vi "TRNPRPdll.vi"(8 "error in (no error)":errorcluster, 11 "Inputs":cluster{"t":dbl, "D":dbl, "z":dbl[]}) -> (0 "error out":errorcluster, 3 "Outputs":T1)   [LabVIEW 2015]
doc: "subroutine TRNPRPdll(t, D, z, eta, tcx, ierr, herr, herr_length)\n\nCompute the transport properties thermal conductivity and viscosity as functions of temperature, density, and\ncomposition.\n\n*** Warning *** Do NOT call this routine for two-phase states, otherwise it will return a metastable state if\nnear the phase boundary or complete nonsense at other conditions. The value of q that is returned from the flash\nroutines will indicate a two phase state by returning a value between 0 and 1. In such a situation, the transport\nproperties can only be calculated for the saturated liquid and vapor states. For example, when calling PHFLSH:\ncall subroutine PHFLSH (P,h,z,T,D,Dl,Dv,x,y,q,e,s,Cv,Cp,w,ierr,herr) If q>0 and q<1, then values of the liquid\ncompositions will be returned in the x and y arrays, and the transport properties of the liquid and vapor states can\nbe calculated as such: call TRNPRP (T,Dl,x,etaliq,tcxliq,ierr,herr) call TRNPRP (T,Dv,y,etavap,tcxvap,ierr,herr)\n\nINPUTS:\nt -- Temperature [K]\nD -- Molar density [mol/L]\nz -- Composition array (array of mole fractions)\n\nOUTPUTS:\neta -- Viscosity [uPa-s]\ntcx -- Thermal conductivity [W/m-K]\nierr -- Error flag: 0 - Successful \n 502 - Unknown viscosity or thermal conductivity model specified \n 503 - One or more inputs are out of bounds for the ECS model \n 504 - Inputs to the vis. and th. cond. correlations are out 2of range \n 540 - Transport equations are not available for one or more of the fluids \n 541 - Transport equations are not available for mixtures with water at molar concentrations greater than 5% \n 542 - Transport equations are not available for mixtures with alcohols \n 543 - Transport equations are not available for the ammonia/water mixture \n -508 - Invalid region for viscosity of reference fluid 1 \n -558 - 2-D Newton-Raphson method for conformal temperature and density did not converge \n -560 - Pure fluid is exactly at the critical point; thermal conductivity is infinite \n 561 - Pure fluid correlation produced an erroneous value for either viscosity or thermal conductivity \n 5## - One or more inputs to the thermal conductivity correlation are out of range; results may be in error \n 5## - One or more inputs to the viscosity correlation are out of range; results may be in error \n 5## - Pure fluid correlation out of range; attempted to use ECS method\nherr -- Error string (character*255)\nherr_length -- length of variable herr (default: 255)"
uses:
  REFPROP.dll
panel:
  # "REFPROP-TRNPRPdll.vi"
  # "void  TRNPRPdll(double *t, double *D, double *z, double *eta, double *tcx, int32_t *ierr, CStr herr, int32_t herr_length)"
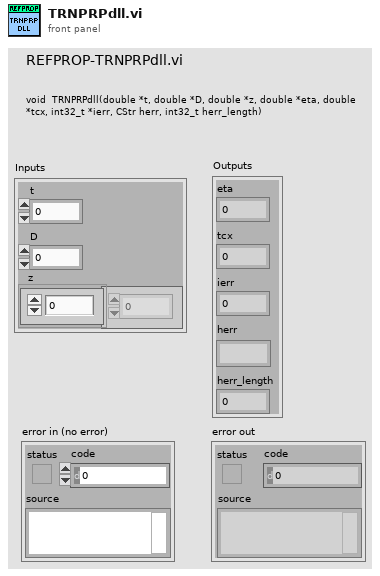
[diagram p1: front panel]
types:
  T1 = cluster{"eta":dbl, "tcx":dbl, "ierr":i32, "herr":string, "herr_length":i32}
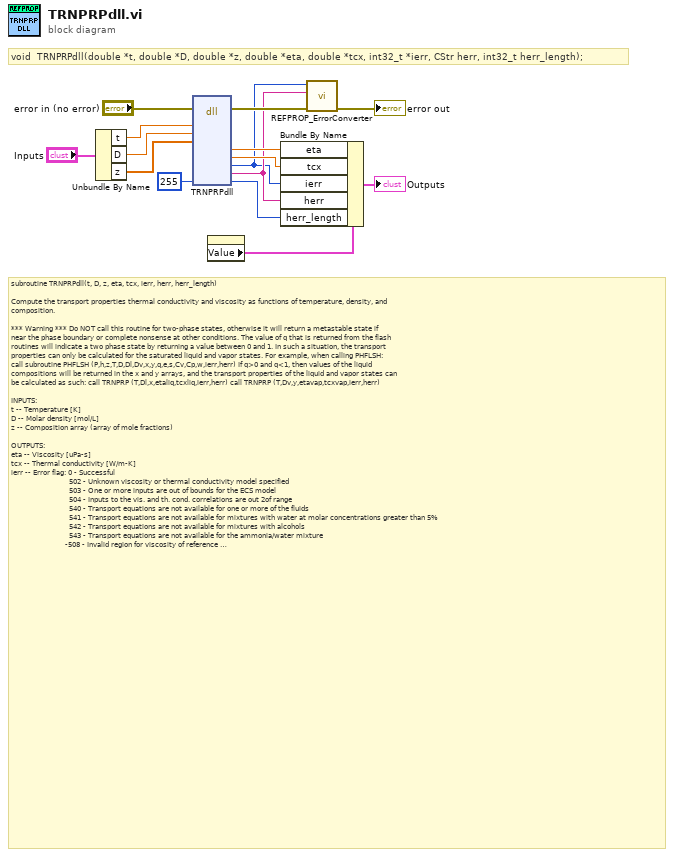
[diagram p0: block diagram]
diagram:
  # "void  TRNPRPdll(double *t, double *D, double *z, double *eta, double *tcx, int32_t *ierr, CStr herr, int32_t herr_length);"
  # "subroutine TRNPRPdll(t, D, z, eta, tcx, ierr, herr, herr_length)\n\nCompute the transport properties thermal conductivity and viscosity as functions of temperature, density, and\ncomposition.\n\n*** Warning *** Do NOT call this routine for two-phase states, otherwise it will return a metastable state if\nnear the phase boundary or complete nonsense at other conditions. The value of q that is returned from the flash\nroutines will indicate a two phase state by returning a value between 0 and 1. In such a situation, the transport\nproperties can only be calculated for the saturated liquid and vapor states. For example, when calling PHFLSH:\ncall subroutine PHFLSH (P,h,z,T,D,Dl,Dv,x,y,q,e,s,Cv,Cp,w,ierr,herr) If q>0 and q<1, then values of the liquid\ncompositions will be returned in the x and y arrays, and the transport properties of the liquid and vapor states can\nbe calculated as such: call TRNPRP (T,Dl,x,etaliq,tcxliq,ierr,herr) call TRNPRP (T,Dv,y,etavap,tcxvap,ierr,herr)\n\nINPUTS:\nt -- Temperature [K]\nD -- Molar density [mol/L]\nz -- Composition array (array of mole fractions)\n\nOUTPUTS:\neta -- Viscosity [uPa-s]\ntcx -- Thermal conductivity [W/m-K]\nierr -- Error flag: 0 - Successful \n                             502 - Unknown viscosity or thermal conductivity model specified \n                             503 - One or more inputs are out of bounds for the ECS model \n                             504 - Inputs to the vis. and th. cond. correlations are out 2of range \n                             540 - Transport equations are not available for one or more of the fluids \n                             541 - Transport equations are not available for mixtures with water at molar concentrations greater than 5% \n                             542 - Transport equations are not available for mixtures with alcohols \n                             543 - Transport equations are not available for the ammonia/water mixture \n                           -508 - Invalid region for viscosity of reference fluid 1 \n                           -558 - 2-D Newton-Raphson method for conformal temperature and density did not converge \n                           -560 - Pure fluid is exactly at the critical point; thermal conductivity is infinite \n                             561 - Pure fluid correlation produced an erroneous value for either viscosity or thermal conductivity \n                             5## - One or more inputs to the thermal conductivity correlation are out of range; results may be in error \n                             5## - One or more inputs to the viscosity correlation are out of range; results may be in error \n                             5## - Pure fluid correlation out of range; attempted to use ECS method\nherr -- Error string (character*255)\nherr_length -- length of variable herr (default: 255)"
  n1 = Unbundle By Name("Inputs") -> ("t"=w10:dbl, "D"=w9:dbl, "z"=w8:dbl[])
  n2 = dll-call lib="C:/Users/lauria/Desktop/REFPROP 10 LabVIEW Wrapper BETA/REFPROP/REFPROP.*" fn="TRNPRPdll"(error in="error in (no error)", "t"=w10, "D"=w9, "z"=w8, "herr_length"=255) -> (error out=w15:errorcluster, "eta"=w6:dbl, "tcx"=w5:dbl, "ierr"=w1:i32, "herr"=w2:string, "herr_length"=w4:i32)  [unwired: 10 in, 1 out]
  n3 = property on="Outputs" class="Clust (strict)"() -> ("Value"=w7:T1)  [unwired: 2 in, 2 out]
  n4 = Bundle By Name(cluster=w7, "eta"=w6, "tcx"=w5, "ierr"=w1, "herr"=w2, "herr_length"=w4) -> (→"Outputs":T1)
  n5 = call "REFPROP_ErrorConverter.vi"("error in (no error)"=w15, "Error Message"=w2, "Error Code"=w1) -> ("error out"=→"error out":errorcluster)  [unwired: 8 in]
